vi "Test matching.vi"() -> ()   [LabVIEW 2015]
uses:
  Name type and data.ctl
  Device/Device type.ctl
  Instruments/Neocera/Neocera LTC-21.lvclass
  Instruments/Oxford/ITC503/ITC 503.lvclass
  Device/Write Name.vi
panel:
  out "Matching pairs":T1(array[cluster])
  in  "Names and data":T2[](array[typedef])=[{"Front Panel Data"=variant, "Device type"=enum."Neocera 21", "Name"="Neocera (21)"}, {"Front Panel Data"=variant, "Device type"=enum."ITC503", "Name"="ITC503 (18)"}, {"Front Panel Data"=variant, "Device type"=enum."Neocera 21", "Name"="Neocera (15)"}]
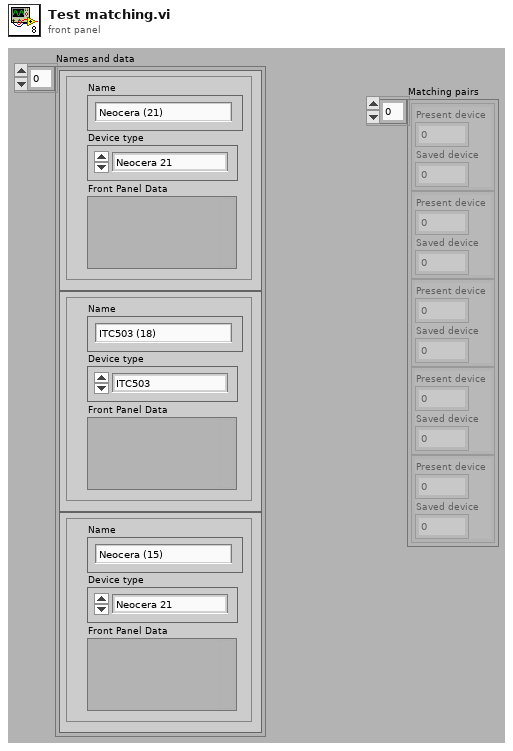
[diagram p1: front panel]
types:
  T1 = cluster{"Present device":i32, "Saved device":i32}[]
  T2 = typedef "Name type and data.ctl" = cluster{"Front Panel Data":variant, "Device type":T3, "Name":string}
  T3 = typedef "Device type.ctl" = enum16{"NONE", "Neocera 21", "LakeShore 335", "LakeShore 340", "LkShr 340 chA&B", "LakeShore 370", "SRS 850", "SRS 830", "LR 700", "EG&G 5302", "EG&G 7260", "EG&G 7280", "AH 2500", "Keithley meter", "Keithley electrometer", "Keithley 182", "HP 5385", "HP 53181", "HP 53132", "ITC503", "IPS120", "Oxford Mercury IPS", "Oxford PS", "Test", "DC Facility Magnet", "Cryomagnetics PS", "Keithley 2400", "Keithley current source", "Cryo-Con 22C", "HP87NN", "HP4395A"}
  T4 = cluster{"Saved device":i32, "Present device":i32}[]
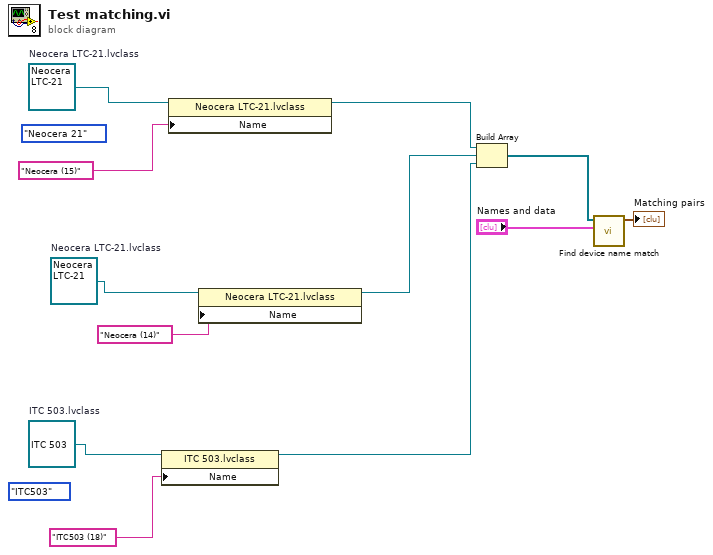
[diagram p0: block diagram]
diagram:
  (unwired) Device_type."ITC503" ("Device type")
  w4 = refnum<class "ITC 503.lvclass"> refnum  # ITC 503.lvclass
  w8 = refnum<class "Neocera LTC-21.lvclass"> refnum  # Neocera LTC-21.lvclass
  (unwired) Device_type."Neocera 21" ("Device type")
  w11 = refnum<class "Neocera LTC-21.lvclass"> refnum  # Neocera LTC-21.lvclass
  n1 = property class="ITC 503.lvclass"(reference=w4, "Name"="ITC503 (18)") -> (reference out=w2:refnum<class "ITC 503.lvclass">)  [unwired: 1 in, 1 out]
  n2 = property class="Neocera LTC-21.lvclass"(reference=w11, "Name"="Neocera (15)") -> (reference out=w7:refnum<class "Neocera LTC-21.lvclass">)  [unwired: 1 in, 1 out]
  n3 = property class="Neocera LTC-21.lvclass"(reference=w8, "Name"="Neocera (14)") -> (reference out=w6:refnum<class "Neocera LTC-21.lvclass">)  [unwired: 1 in, 1 out]
  n4 = Build Array(w7, w6, w2) -> (w5:refnum<class "Temperature controller.lvclass">[])
  n5 = call "Find device name match.vi"("Saved names and data"="Names and data", "Device list"=w5) -> ("Matching pairs"=→"Matching pairs":T4)  [unwired: 8 in, 1 out]
